vi "PXI Sensor Task.vi"(8 "error in":errorcluster) -> (0 "error out":errorcluster, 3 "task out":refnum<k21>)   [LabVIEW 2014]
uses:
  <vilib>/DAQmx/create/channels.llb/DAQmx Create Channel (DI-Digital Input).vi
  <resource>/objmgr/daqmx.rc
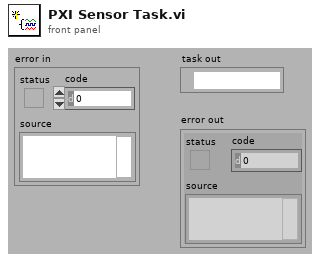
[diagram p1: front panel]
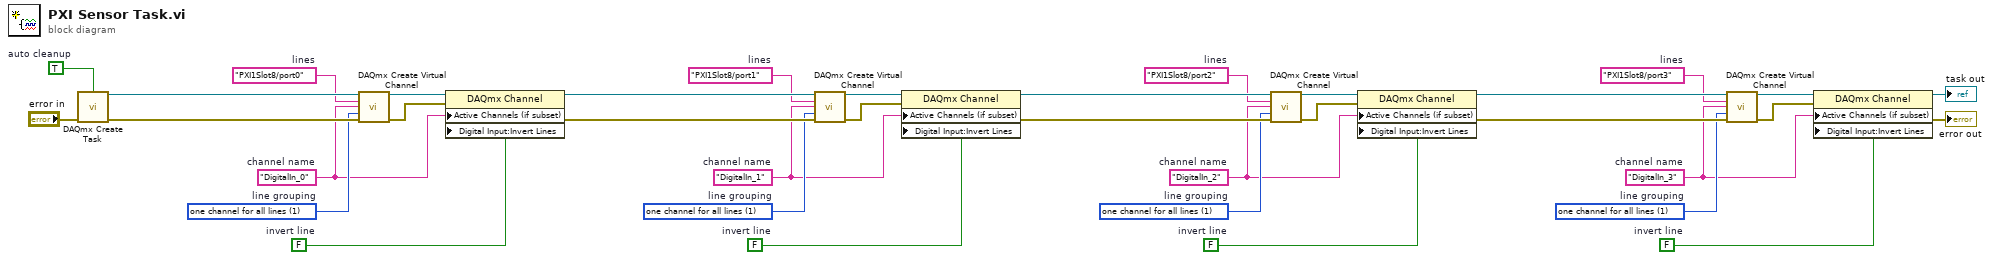
[diagram p0: block diagram]
diagram:
  w2 = FALSE  # invert line
  w7 = 1 items=["one channel for each line", "one channel for all lines"]  # line grouping
  w1 = "DigitalIn_3"  # channel name
  w8 = "PXI1Slot8/port3"  # lines
  w11 = FALSE  # invert line
  w15 = 1 items=["one channel for each line", "one channel for all lines"]  # line grouping
  w10 = "DigitalIn_2"  # channel name
  w16 = "PXI1Slot8/port2"  # lines
  w19 = FALSE  # invert line
  w23 = 1 items=["one channel for each line", "one channel for all lines"]  # line grouping
  w18 = "DigitalIn_1"  # channel name
  w24 = "PXI1Slot8/port1"  # lines
  w27 = FALSE  # invert line
  w31 = 1 items=["one channel for each line", "one channel for all lines"]  # line grouping
  w26 = "DigitalIn_0"  # channel name
  w32 = "PXI1Slot8/port0"  # lines
  w34 = TRUE  # auto cleanup
  n1 = call <vilib>:"DAQmx Create Task.vi"("auto cleanup"=w34, "error in"="error in") -> ("task out"=w33:refnum<k21>, "error out"=w35:errorcluster)  [unwired: 12 in]
  n2 = call-poly <vilib>:"DAQmx Create Virtual Channel.vi"("task in"=w33, "lines"=w32, "name to assign"=w26, "line grouping"=w31, "error in"=w35) -> ("task out"=w30:refnum<k21>, "error out"=w29:errorcluster)  [unwired: 9 in]
  n3 = property class="DAQmx Channel"(reference=w30, error in=w29, "Active Channels (if subset)"=w26, "Digital Input:Invert Lines"=w27) -> (reference out=w25:refnum<k21>, error out=w28:errorcluster)
  n4 = call-poly <vilib>:"DAQmx Create Virtual Channel.vi"("task in"=w25, "lines"=w24, "name to assign"=w18, "line grouping"=w23, "error in"=w28) -> ("task out"=w22:refnum<k21>, "error out"=w21:errorcluster)  [unwired: 9 in]
  n5 = property class="DAQmx Channel"(reference=w22, error in=w21, "Active Channels (if subset)"=w18, "Digital Input:Invert Lines"=w19) -> (reference out=w17:refnum<k21>, error out=w20:errorcluster)
  n6 = call-poly <vilib>:"DAQmx Create Virtual Channel.vi"("task in"=w17, "lines"=w16, "name to assign"=w10, "line grouping"=w15, "error in"=w20) -> ("task out"=w14:refnum<k21>, "error out"=w13:errorcluster)  [unwired: 9 in]
  n7 = property class="DAQmx Channel"(reference=w14, error in=w13, "Active Channels (if subset)"=w10, "Digital Input:Invert Lines"=w11) -> (reference out=w9:refnum<k21>, error out=w12:errorcluster)
  n8 = call-poly <vilib>:"DAQmx Create Virtual Channel.vi"("task in"=w9, "lines"=w8, "name to assign"=w1, "line grouping"=w7, "error in"=w12) -> ("task out"=w6:refnum<k21>, "error out"=w5:errorcluster)  [unwired: 9 in]
  n9 = property class="DAQmx Channel"(reference=w6, error in=w5, "Active Channels (if subset)"=w1, "Digital Input:Invert Lines"=w2) -> (reference out=→"task out":refnum<k21>, error out=→"error out":errorcluster)
